vi "提取轮廓行列(子VI).vi"(6 "reference 3":refnum<vi>, 7 "reference":refnum<vi>, 9 "reference 4":refnum<vi>, 10 "reference 2":refnum<vi>, 11 "引用句柄输入":T1) -> (1 "车尾列":u8[](array[numeric]), 2 "车头列":u8[](array[numeric]), 3 "车顶行":u8[](array[numeric]), 4 "车底行":u8[](array[numeric]))   [LabVIEW 2012]
uses:
  <vilib>/vision/Image Controls.llb/IMAQ Image.ctl
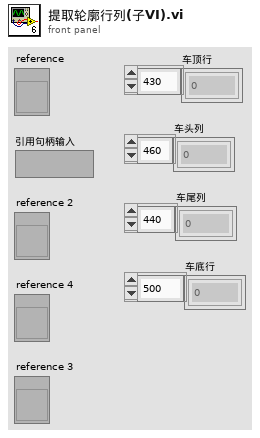
[diagram p1: front panel]
types:
  T1 = typedef "IMAQ Image.ctl" = refnum<image>
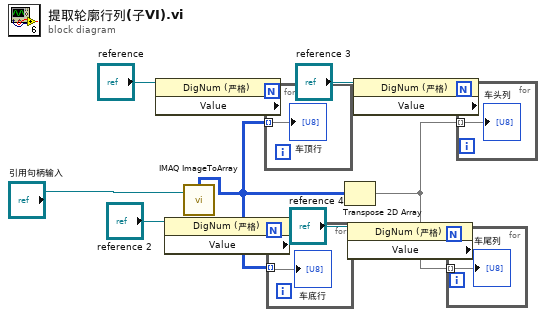
[diagram p0: block diagram]
diagram:
  n1 = property class="DigNum (严格)"(reference="reference") -> ("Value"=w10:i32)  [unwired: 1 in, 2 out]
  n2 = property class="DigNum (严格)"(reference="reference 2") -> ("Value"=w6:i32)  [unwired: 1 in, 2 out]
  n3 = call "IMAQ ImageToArray"("Image"="引用句柄输入") -> ("Image Pixels (U8)"=w9:u8[][])  [unwired: 3 in, 4 out]
  n4 = for {
    N: w10 -> [_]
    tunnel: w9 -> [w12] mode=indexing
    "车顶行" <- w12
  }
  n5 = for {
    N: w6 -> [_]
    tunnel: w9 -> [w13] mode=indexing
    "车底行" <- w13
  }
  n6 = Transpose 2D Array(2D array=w9) -> (transposed array=w8:u8[][])
  n7 = property class="DigNum (严格)"(reference="reference 4") -> ("Value"=w7:i32)  [unwired: 1 in, 2 out]
  n8 = property class="DigNum (严格)"(reference="reference 3") -> ("Value"=w11:i32)  [unwired: 1 in, 2 out]
  n9 = for {
    N: w7 -> [_]
    tunnel: w8 -> [w14] mode=indexing
    "车尾列" <- w14
  }
  n10 = for {
    N: w11 -> [_]
    tunnel: w8 -> [w15] mode=indexing
    "车头列" <- w15
  }
